vi "sensitivity.vi"(1 "input":dbl format="%#_13g", 2 "Sensitivity":dbl=0.26 format="%#_13g") -> (0 "output":dbl)   [LabVIEW 2017]
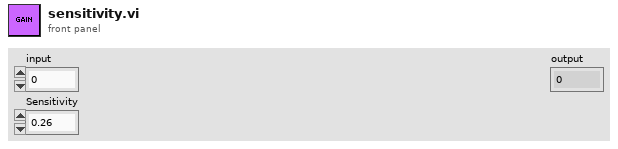
[diagram p1: front panel]
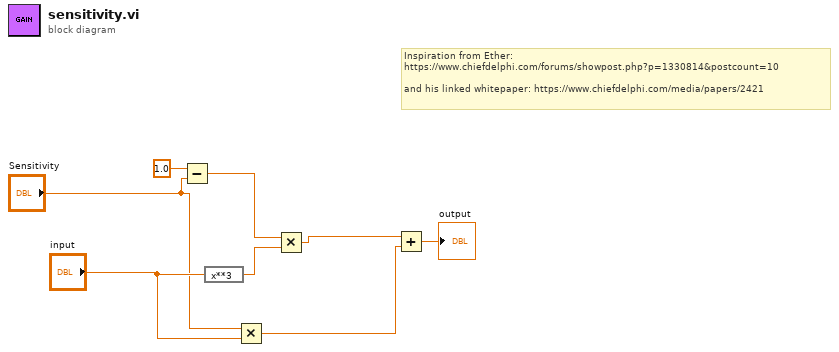
[diagram p0: block diagram]
diagram:
  # "Inspiration from Ether:\nhttps://www.chiefdelphi.com/forums/showpost.php?p=1330814&postcount=10\n\nand his linked whitepaper: https://www.chiefdelphi.com/media/papers/2421"
  n1 = Subtract(x=1.0, y="Sensitivity") -> (x-y=w4:dbl)
  n2 = expression code="x**3"("input") -> (w8:dbl)
  n3 = Multiply(x="Sensitivity", y="input") -> (x*y=w1:dbl)
  n4 = Multiply(x=w4, y=w8) -> (x*y=w2:dbl)
  n5 = Add(x=w2, y=w1) -> (x+y=→"output":dbl)
